vi "todo.vi"() -> ()   [LabVIEW 2019]
uses:
  <userlib>/Nanonis Prog Interface/Nanonis Prog Interface.lvlib
panel:
  out "I-gain":sgl format="%#_6p"
  out "Time constant (s)":sgl format="%#_6p"
  out "P-gain":sgl format="%#_6p"
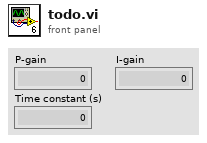
[diagram p1: front panel]
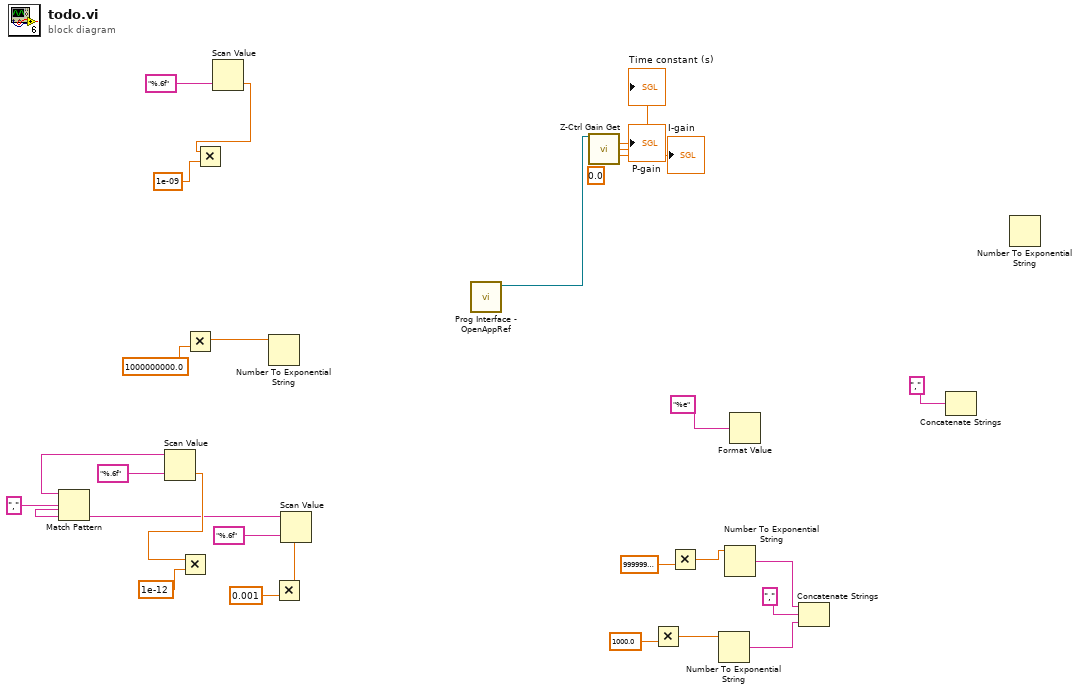
[diagram p0: block diagram]
diagram:
  (unwired) sgl 0.0 ("P-gain")
  n1 = Match Pattern(regular expression=",") -> (string=w16:string, before substring=w15:string, after substring=w12:string)  [unwired: 1 in, 2 out]
  n2 = Scan Value(string=w15, format string="%.6f") -> (value=w18:dbl)  [unwired: 1 in, 1 out]
  n3 = Multiply(x=w18, y=1e-12) -> (x*y=w14:dbl)
  n4 = Multiply(y=1000000000.0) -> (x=w22:dbl, x*y=w21:dbl)
  n5 = Scan Value(format string="%.6f") -> (string=w27:string, value=w25:dbl)  [unwired: 1 in, 1 out]
  n6 = Multiply(x=w25, y=1e-09) -> (x*y=w24:dbl)
  n7 = Number To Exponential String(number=w21) -> ()  [unwired: 3 in, 1 out]
  n8 = Scan Value(string=w12, format string="%.6f") -> (value=w9:dbl)  [unwired: 1 in, 1 out]
  n9 = Multiply(x=w9, y=0.001) -> (x*y=w11:dbl)
  n10 = call <userlib>:"Prog Interface - OpenAppRef.vi"() -> ("Application reference"=w34:refnum<vi>)  [unwired: 6 in, 1 out]
  n11 = call <userlib>:"Z-Ctrl Gain Get.vi"("Application ref in"=w34) -> ("P-gain"=→"P-gain":sgl, "Time constant (s)"=→"Time constant (s)":sgl, "I-gain"=→"I-gain":sgl)  [unwired: 10 in, 2 out]
  n12 = Multiply(y=sgl 1000.0) -> (x*y=w7:sgl)  [unwired: 1 in]
  n13 = Multiply(y=sgl 1000000000000.0) -> (x=w6:sgl, x*y=w8:sgl)
  n14 = Number To Exponential String(number=w7) -> (E-format string=w1:string)  [unwired: 3 in]
  n15 = Number To Exponential String(number=w8) -> (E-format string=w2:string)  [unwired: 3 in]
  n16 = Format Value(format string="%e") -> ()  [unwired: 2 in, 1 out]
  n17 = Concatenate Strings(w2, "," ("string"), w1) -> ()  [unwired: 1 out]
  n18 = Concatenate Strings("," ("string")) -> ()  [unwired: 2 in, 1 out]
  n19 = Number To Exponential String() -> ()  [unwired: 4 in, 1 out]
